vi "Select Greater_nevstop.vi"(0 "A":dbl, 3 "B":dbl) -> (5 "Lesser":dbl)   [LabVIEW 2017, in "csm-tool-support.lvlib"]
doc: "### Select Greater_nevstop.vi\n\n-- <b>Controls</b> --\n- <b>A</b>:\n- <b>B</b>:\n\n-- <b>Indicators</b> --\n- <b>lesser</b>:"
uses:
  csm-tool-support.lvlib
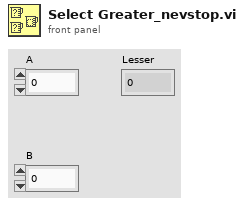
[diagram p1: front panel]
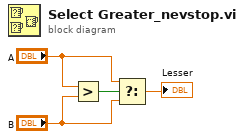
[diagram p0: block diagram]
diagram:
  n1 = Greater?(x="A", y="B") -> (0:w4:bool)
  n2 = Select(t="A", s=w4, f="B") -> (s? t:f=→"Lesser":dbl)
